vi "Double Timestamp to Unix ns (Array).vi"(3 "Timestamp":dbl[](array[numeric])) -> (1 "unix ns":i64[](array[numeric]))   [LabVIEW 2020, in "Vecto.lvlib"]
uses:
  Vecto.lvlib
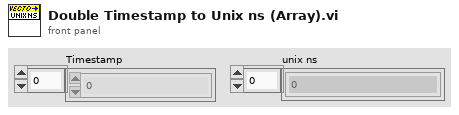
[diagram p1: front panel]
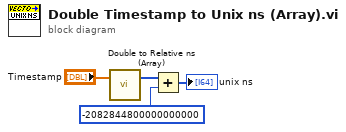
[diagram p0: block diagram]
diagram:
  n1 = call "Double to Relative ns (Array).vi"("Double"="Timestamp") -> ("Relative ns"=w1:i64[])  [unwired: 2 in]
  n2 = Add(x=w1, y=i64 -2082844800000000000) -> (x+y=→"unix ns":i64[])
